vi "Pockels Cal_Save.vi"(11 "Pockels Cal table (inc. headers & info)":string[][](array[string])) -> (0 "error out":errorcluster, 3 "Updated existing file?":bool)   [LabVIEW 2020]
uses:
  Typedefs/Which path.ctl
  gl_Calibration globals.vi
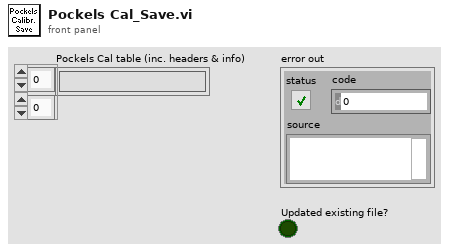
[diagram p1: front panel]
types:
  T1 = typedef "Which path.ctl" = enum16{"Configuration Files", "Calibration Files", "Images", "Setup.ini", "Loaded User profile.ini", "User's-Previous session.ini", "New user profile.ini", "Selected User profile.ini", "User profiles folder", "Power meter scaling.txt", "FOV Cal.ini", "Calibration.ini"}
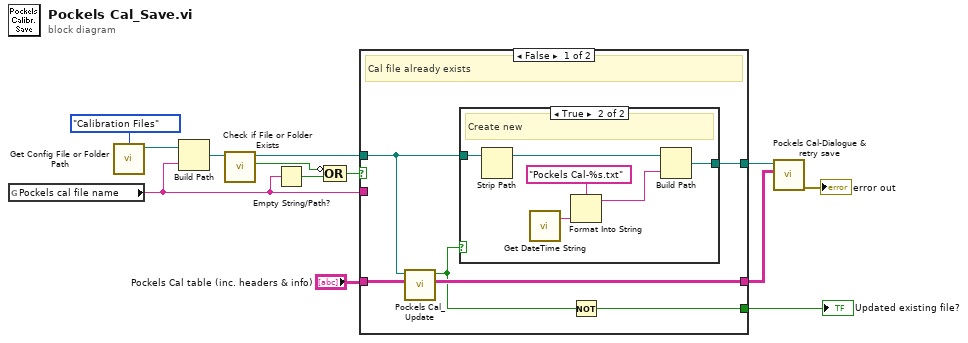
[diagram p0: block diagram]
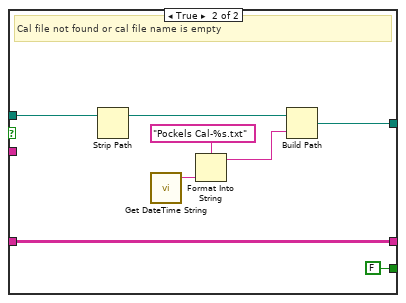
[diagram p3: hidden frame]
diagram:
  n1 = global read "gl_Calibration globals.vi" "Pockels cal file name"() -> (w7:string)
  n2 = call "Get Config File or Folder Path.vi"("Which file or folder?"=Which_path."Calibration Files" ("Which path?")) -> ("File Path"=w12:path)  [unwired: 8 in, 2 out]
  n3 = Build Path(base path=w12, name or relative path=w7) -> (appended path=w10:path)
  n4 = call <vilib>:"Check if File or Folder Exists.vi"("path"=w10) -> ("file or folder exists?"=w6:bool, "dup path"=w9:path)  [unwired: 8 in, 1 out]
  n5 = Empty String/Path?(string/path=w7) -> (empty?=w4:bool)
  n6 = Compound Arithmetic op=OR(invert w6, w4) -> (w3:bool)
  n7 = case shown="False" w3 {
    tunnel: "Pockels Cal table (inc. headers & info)" -> [w19 w32]
    tunnel: w9 -> [w16 w31]
    tunnel: w7 -> [_ _]
    tunnel: [w17 w29] -> w2
    tunnel: [w18 w32] -> w5
    tunnel: [w14 FALSE] -> w1
    frame False {
      # "Cal file already exists"
      n8 = call "Pockels Cal_Update.vi"("New cal section"=w19, "Existing pockels Cal file path"=w16) -> ("Cal file strings"=w18:string[][], "Create new"=w15:bool)  [unwired: 8 in]
      n9 = case shown="True" w15 {
        tunnel: [w20 w21] -> w17
        tunnel: w16 -> [w20 w24]
        frame False {
          # "Update existing"
        }
        frame True {
          # "Create new"
          n10 = Strip Path(path=w24) -> (stripped path=w22:path)  [unwired: 1 out]
          n11 = call <userlib>:"Get DateTime String.vi"() -> ("date/time string"=w26:string)  [unwired: 10 in, 1 out]
          n12 = Format Into String(format string="Pockels Cal-%s.txt", w26) -> (resulting string=w23:string)  [unwired: 2 in, 1 out]
          n13 = Build Path(base path=w22, name or relative path=w23) -> (appended path=w21:path)
        }
      }
      n14 = Not(x=w15) -> (.not. x?=w14:bool)
    }
    frame True {
      # "Cal file not found or cal file name is empty"
      n15 = Strip Path(path=w31) -> (stripped path=w30:path)  [unwired: 1 out]
      n16 = call <userlib>:"Get DateTime String.vi"() -> ("date/time string"=w34:string)  [unwired: 10 in, 1 out]
      n17 = Format Into String(format string="Pockels Cal-%s.txt", w34) -> (resulting string=w28:string)  [unwired: 2 in, 1 out]
      n18 = Build Path(base path=w30, name or relative path=w28) -> (appended path=w29:path)
    }
  }
  "Updated existing file?" <- w1
  n19 = call "Pockels Cal-Dialogue & retry save.vi"("Pockels Cal table"=w5, "Pockels cal file path"=w2) -> ("error out"=→"error out":errorcluster)  [unwired: 9 in]
